vi "multiple VI Decode.vi"() -> ()   [LabVIEW 2016]
uses:
  Single VI Decode.vi
panel:
  out "Slide":i32(slide) scale=0.0..13.0
  in  "Folder Path":path
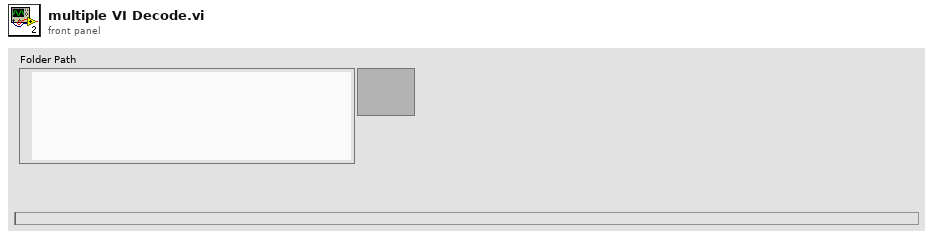
[diagram p1: front panel]
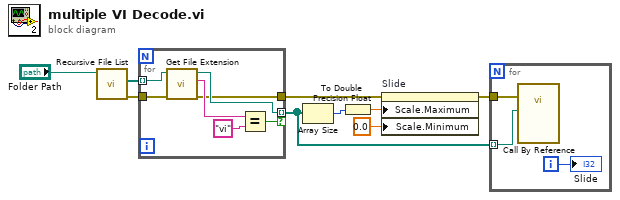
[diagram p0: block diagram]
diagram:
  n1 = call <vilib>:"Recursive File List.vi"("Folder Path"="Folder Path") -> ("error out"=w7:errorcluster, "All Files in Dir"=w8:path[])  [unwired: 6 in, 3 out]
  n2 = for {
    tunnel: w8 -> [w16] mode=indexing
    tunnel: w7 -> [w15]
    tunnel: [w12] -> w4 mode=indexing if=w11
    tunnel: [w10] -> w6
    n3 = call <vilib>:"Get File Extension.vi"("error in (no error)"=w15, "file"=w16) -> ("error out"=w10:errorcluster, "lowercase file extension"=w14:string, "dup file"=w12:path)  [unwired: 5 in, 2 out]
    n4 = Equal?(x=w14, y="vi") -> (x = y?=w11:bool)
  }
  n5 = Array Size(array=w4) -> (size(s)=w3:i32)
  n6 = To Double Precision Float(number=w3) -> (double precision float=w2:dbl)
  n7 = property on="Slide" class="Slide (strict)"(error in=w6, "Scale.Maximum"=w2, "Scale.Minimum"=0.0 ("Scale.Range:Minimum")) -> (error out=w5:errorcluster)  [unwired: 1 in, 1 out]
  n8 = for {
    tunnel: w4 -> [w18] mode=indexing
    tunnel: w5 -> [w17]
    i -> [w19]
    n9 = call-by-ref "?"(error in=w17, "filename (use dialog)"=w18) -> ()  [unwired: 12 in, 2 out]
    "Slide" <- w19
  }
